vi "MotorPositionControllerDelete.vi"(8 "error in":errorcluster, 11 "Device In":u64) -> (0 "error out":errorcluster)   [LabVIEW 2012, in "Phidget Motor Position Controller.lvlib"]
doc: "Deletes a Phidget DC Motor"
uses:
  <instrlib>/Phidgets/Phidget Motor Position Controller/Phidget Motor Position Controller.lvlib
  <instrlib>/Phidgets/Phidget Common/Phidget Common.lvlib
  phidget22.dll
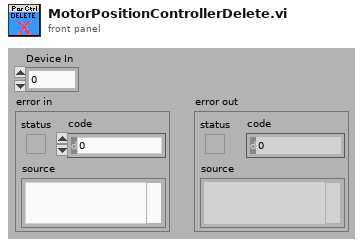
[diagram p1: front panel]
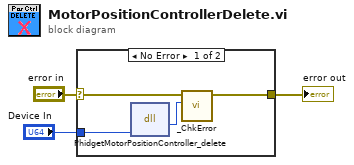
[diagram p0: block diagram]
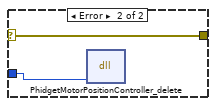
[diagram p2: hidden frame]
diagram:
  n1 = case shown="No Error" "error in" {
    selector: "error in" -> [w5 w9]
    tunnel: [w4 w9] -> w2
    tunnel: "Device In" -> [w6 w8]
    frame No Error {
      n2 = dll-call lib="phidget22.*" fn="PhidgetMotorPositionController_delete"("phid"=w6) -> ("return type"=w7:i32)  [unwired: 4 in, 2 out]
      n3 = call <instrlib>:"_ChkError.vi"("Return Code"=w7, "error in (no error)"=w5) -> ("error out"=w4:errorcluster)  [unwired: 9 in]
    }
    frame Error {
      n4 = dll-call lib="phidget22.*" fn="PhidgetMotorPositionController_delete"("phid"=w8) -> ()  [unwired: 5 in, 2 out]
    }
  }
  "error out" <- w2
